vi "Fetch Measurement (Noise).vi"(0 "VISA resource name":refnum<visa-resource-name>, 1 "Measure Type (0: Zero)":i32(ring) items=["Zero", "One", "Both"], 5 "Source (0: Channel 1)":i32(ring) items=["Channel 1", "Channel 2", "Channel 3", "Channel 4", "Function 1", "Function 2", "Function 3", "Function 4", "Memory 1", "Memory 2", "Memory 3", "Memory 4", "Equalized"], 7 "Units (0: Volt)":i32(ring) items=["Volt", "Unit"], 11 "error in (no error)":errorcluster) -> (4 "VISA resource name out":refnum<visa-resource-name>, 10 "Noise Value":dbl, 15 "error out":errorcluster)   [LabVIEW 2020, in "Agilent 90000 Series.lvlib"]
doc: "Returns the result of a noise measurement.\n\n<B>Note:</B> \nUse this VI only with other low-level VIs. The high-level VIs automatically incorporate this functionality. This VI does not check the instrument status."
uses:
  Agilent 90000 Series.lvlib
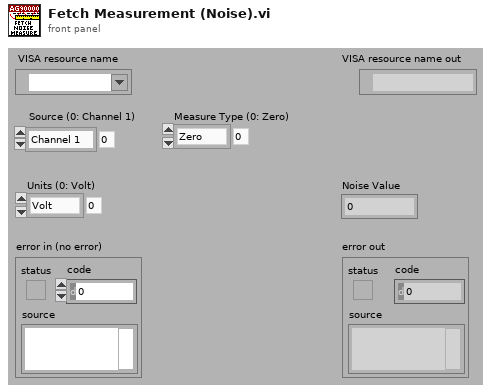
[diagram p1: front panel]
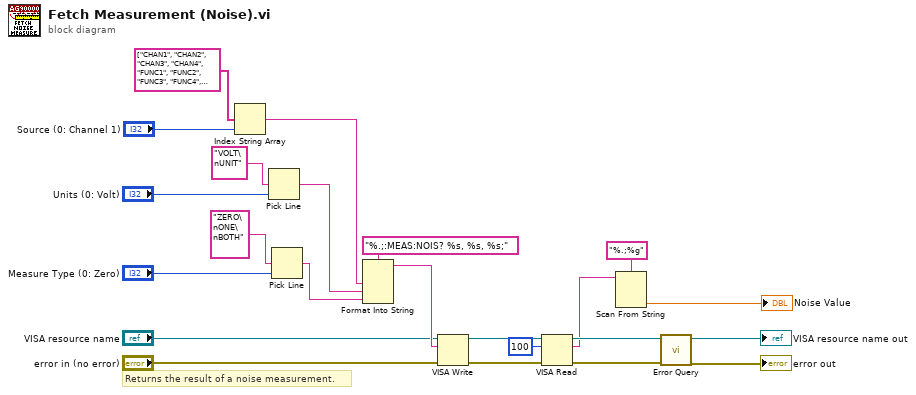
[diagram p0: block diagram]
diagram:
  # "Returns the result of a noise measurement."
  n1 = Index String Array(1:"Source (0: Channel 1)", 2:string[] ["CHAN1", "CHAN2", "CHAN3", "CHAN4", "FUNC1", "FUNC2", "FUNC3", "FUNC4", "WMEM1", "WMEM2", "WMEM3", "WMEM4", "EQU"]) -> (0:w9:string)  [unwired: 1 out]
  n2 = Pick Line(multi-line string="VOLT\nUNIT", line index="Units (0: Volt)") -> (output string=w18:string)  [unwired: 1 out]
  n3 = Pick Line(multi-line string="ZERO\nONE\nBOTH", line index="Measure Type (0: Zero)") -> (output string=w17:string)  [unwired: 1 out]
  n4 = Format Into String(format string="%.;:MEAS:NOIS? %s, %s, %s;", w9, w18, w17) -> (resulting string=w16:string)  [unwired: 2 in, 1 out]
  n5 = VISA Write(VISA resource name="VISA resource name", write buffer=w16, error in (no error)="error in (no error)") -> (VISA resource name out=w8:refnum<visa-resource-name>, error out=w7:errorcluster)  [unwired: 1 out]
  n6 = VISA Read(VISA resource name=w8, byte count=u32 100, error in (no error)=w7) -> (VISA resource name out=w6:refnum<visa-resource-name>, read buffer=w1:string, error out=w5:errorcluster)  [unwired: 1 out]
  n7 = Scan From String(format string="%.;%g", input string=w1) -> (output 1=→"Noise Value":dbl)  [unwired: 2 in, 4 out]
  n8 = call "Error Query.vi"("error in (no error)"=w5, "VISA resource name"=w6) -> ("error out"=→"error out":errorcluster, "VISA resource name out"=→"VISA resource name out":refnum<visa-resource-name>)  [unwired: 8 out]
